vi "Vision subvi.vi"(8 "error in (no error)":errorcluster, 11 "Image Src":T1) -> (0 "error out 2":errorcluster, 2 "element 2":T2, 3 "Image Out 2":T1(plugin-control))   [LabVIEW 2018]
uses:
  <vilib>/vision/Image Controls.llb/IMAQ Image.ctl
  <vilib>/vision/NI_Vision_Development_Module.lvlib
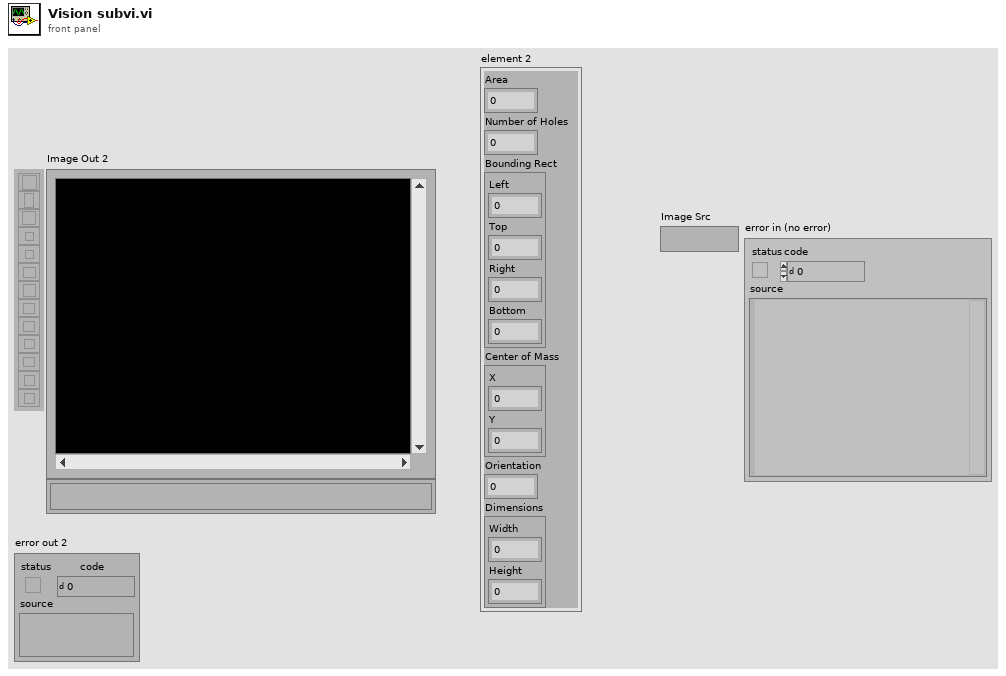
[diagram p1: front panel]
types:
  T1 = typedef "IMAQ Image.ctl" = refnum<image>
  T2 = cluster{"Area":dbl, "Number of Holes":dbl, "Bounding Rect":cluster{"Left":dbl, "Top":dbl, "Right":dbl, "Bottom":dbl}, "Center of Mass":cluster{"X":dbl, "Y":dbl}, "Orientation":dbl, "Dimensions":cluster{"Width":dbl, "Height":dbl}}
  T3 = enum32{"AutoM", "Close", "Dilate", "Erode", "Gradient", "Gradient out", "Gradient in", "Hit miss", "Open", "PClose", "POpen", "Thick", "Thin"}
  T4 = typedef "Particle Parameters" = i32
  T5 = cluster{"Measurement Parameter":T4, "Range Lower Value":dbl, "Range Upper Value":dbl, "Range":bool, "Measurement Type":bool}[]
  T6 = cluster{"Brightness":sgl, "Contrast":sgl, "Gamma":sgl}
  T7 = cluster{"Measurement Parameter":i32, "Range Lower Value":dbl, "Range Upper Value":dbl, "Range":bool, "Measurement Type":bool}[]
  T8 = cluster{"Area":dbl, "Number of Holes":dbl, "Bounding Rect":cluster{"Left":dbl, "Top":dbl, "Right":dbl, "Bottom":dbl}, "Center of Mass":cluster{"X":dbl, "Y":dbl}, "Orientation":dbl, "Dimensions":cluster{"Width":dbl, "Height":dbl}}[]
  T9 = cluster{"Left":dbl, "Top":dbl, "Right":dbl, "Bottom":dbl}
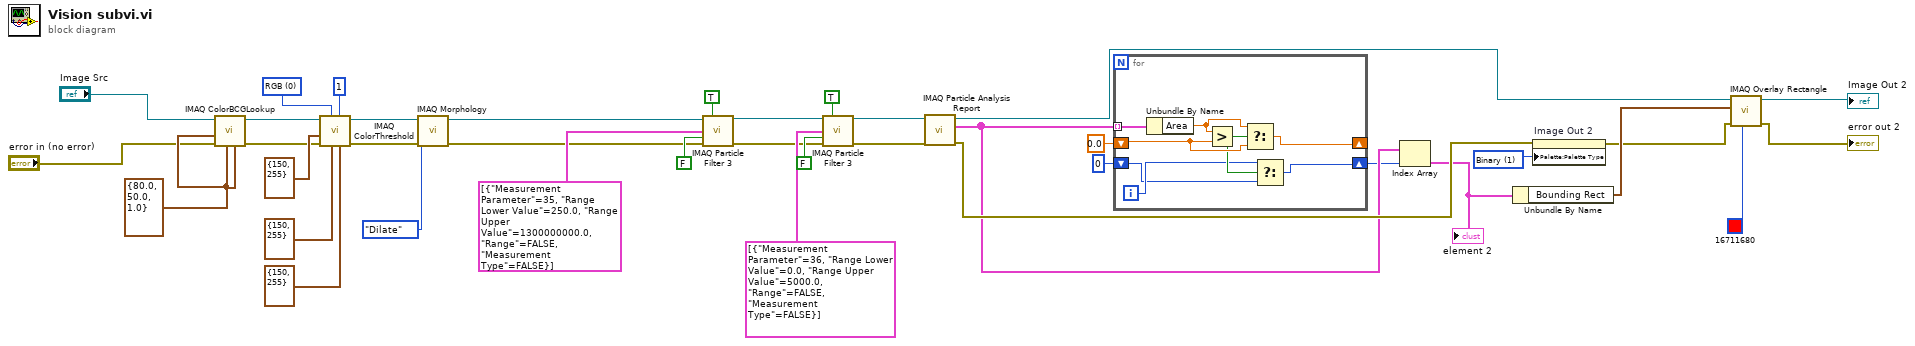
[diagram p0: block diagram]
diagram:
  w28 = T6 {"Brightness"=80.0, "Contrast"=50.0, "Gamma"=1.0} ("Green BCG Values")
  w30 = u32 1 items=["Grayscale", "Binary", "Gradient", "Rainbow", "Temperature", "User Defined", "Binary 16 Bit", "Gradient 16 Bit", "Rainbow 16 Bit", "Temperature 16 Bit", "User Defined 16 Bit"] ("Palette Type")
  w37 = u16 0 items=["RGB", "HSL", "HSV", "HSI"] ("Color Mode")
  n1 = call "IMAQ ColorBCGLookup"("Blue BCG Values"=w28, "Green BCG Values"=w28, "error in (no error)"="error in (no error)", "Red BCG Values"=w28, "Image Src"="Image Src") -> ("error out"=w10:errorcluster, "Image Dst Out"=w9:T1)  [unwired: 2 in, 3 out]
  n2 = call "IMAQ ColorThreshold"("Blue or Luma or Val or Inten Range"=cluster{"Lower value":i32, "Upper value":i32} {"Lower value"=150, "Upper value"=255}, "Replace Value"=1, "Green or Sat Range"=cluster{"Lower value":i32, "Upper value":i32} {"Lower value"=150, "Upper value"=255}, "Color Mode"=w37, "error in (no error)"=w10, "Red or Hue Range"=cluster{"Lower value":i32, "Upper value":i32} {"Lower value"=150, "Upper value"=255}, "Image Src"=w9) -> ("error out"=w2:errorcluster, "Image Dst Out"=w4:T1)  [unwired: 1 in, 2 out]
  n3 = call "IMAQ Morphology"("error in (no error)"=w2, "Operation"=T3."Dilate", "Image Src"=w4) -> ("error out"=w1:errorcluster, "Image Dst Out"=w3:T1)  [unwired: 7 in]
  n4 = call "IMAQ Particle Filter 3"("Image Src"=w3, "Connectivity 4/8 (8)"=TRUE, "Selection Values"=T7 [{"Measurement Parameter"=35, "Range Lower Value"=250.0, "Range Upper Value"=1300000000.0, "Range"=FALSE, "Measurement Type"=FALSE}], "Keep/Remove Particles (F)"=FALSE ("Keep/Remove Particles"), "error in (no error)"=w1) -> ("Image Dst Out"=w7:T1, "error out"=w6:errorcluster)  [unwired: 4 in, 5 out]
  n5 = call "IMAQ Particle Filter 3"("Image Src"=w7, "Connectivity 4/8 (8)"=TRUE, "Selection Values"=T5 [{"Measurement Parameter"=36, "Range Lower Value"=0.0, "Range Upper Value"=5000.0, "Range"=FALSE, "Measurement Type"=FALSE}], "Keep/Remove Particles (F)"=FALSE ("Keep/Remove Particles"), "error in (no error)"=w6) -> ("Image Dst Out"=w13:T1, "error out"=w12:errorcluster)  [unwired: 4 in, 5 out]
  n6 = call "IMAQ Particle Analysis Report"("error in (no error)"=w12, "Image"=w13) -> ("error out"=w25:errorcluster, "Particle Reports (Pixels)"=w24:T8, "Image Out (duplicate)"=w22:T1)  [unwired: 4 in, 3 out]
  n7 = for {
    tunnel: w24 -> [w46] mode=indexing
    shift-right: [w43] -> _
    shift-left: 0.0 ("Area") -> [w44]
    shift-right: [w40] -> w23
    shift-left: 0 -> [w39]
    i -> [w41]
    n8 = Unbundle By Name(w46) -> ("Area"=w45:dbl)
    n9 = Greater?(x=w45, y=w44) -> (0:w42:bool)
    n10 = Select(t=w45, s=w42, f=w44) -> (s? t:f=w43:dbl)
    n11 = Select(t=w41, s=w42, f=w39) -> (s? t:f=w40:i32)
  }
  n12 = Index Array(array=w24, index=w23) -> (element=w19:T2)
  "element 2" <- w19
  n13 = Unbundle By Name(w19) -> ("Bounding Rect"=w18:T9)
  n14 = property on="Image Out 2" class="ImageControl"(error in=w25, "Palette:Palette Type"=w30) -> (error out=w17:errorcluster)  [unwired: 1 in, 1 out]
  n15 = call "IMAQ Overlay Rectangle"("Color"=u32 16711680, "error in (no error)"=w17, "Rectangle"=w18, "Image"=w22) -> ("error out"=→"error out 2":errorcluster, "Image Out"=→"Image Out 2":T1)  [unwired: 6 in]
